vi "WireConnect.vi"(0 "__args":T1) -> (1 "__return":i32, 2 "__errStatus":bool, 3 "__errCode":i32, 4 "__errSource":string)   [LabVIEW 2013]
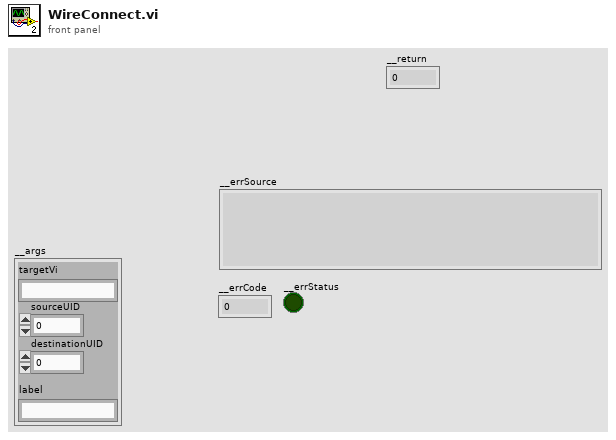
[diagram p1: front panel]
types:
  T1 = cluster{"targetVi":string, "sourceUID":i32, "destinationUID":i32, "label":string}
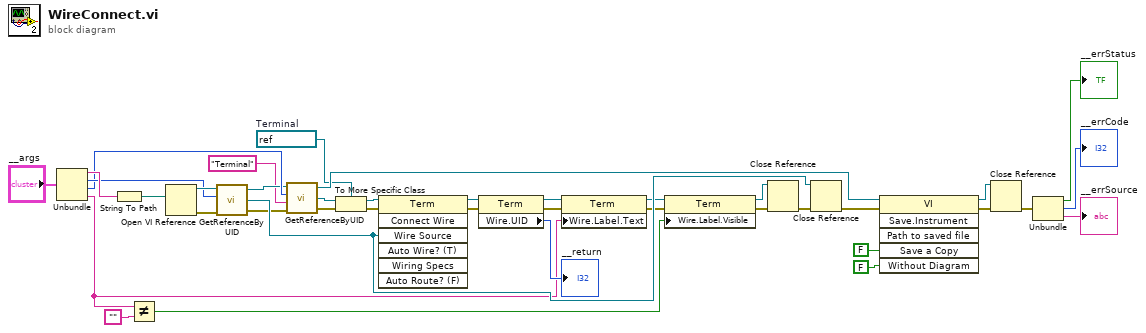
[diagram p0: block diagram]
diagram:
  w11 = refnum<vi> refnum  # Terminal
  n1 = Unbundle("__args") -> ("targetVi"=w28:string, "sourceUID"=w27:i32, "destinationUID"=w26:i32, "label"=w2:string)
  n2 = String To Path(string=w28) -> (path=w35:path)
  n3 = Not Equal?(x=w2, y="") -> (x != y?=w3:bool)
  n4 = Open VI Reference(vi path=w35) -> (vi reference=w34:refnum<vi>, error out=w33:errorcluster)  [unwired: 5 in]
  n5 = call "GetReferenceByUID.vi"("error in (no error)"=w33, "UID"=w27, "targetVI"=w34) -> ("error out"=w13:errorcluster, "refNum"=w14:refnum<vi>, "dup targetVI"=w25:refnum<vi>)  [unwired: 1 in]
  n6 = call "GetReferenceByUID.vi"("error in (no error)"=w13, "objectClass"="Terminal", "UID"=w26, "targetVI"=w25) -> ("error out"=w23:errorcluster, "refNum"=w22:refnum<vi>, "dup targetVI"=w24:refnum<vi>)
  n7 = To More Specific Class(target class=w11, reference=w22, error in=w23) -> (specific class reference=w21:refnum<vi>, error out=w20:errorcluster)
  n8 = invoke class="Term" method="Connect Wire"(reference=w21, error in=w20, "Wire Source"=w14) -> (reference out=w17:refnum<vi>, error out=w15:errorcluster)  [unwired: 4 in, 5 out]
  n9 = property class="Term"(reference=w17, error in=w15) -> (reference out=w9:refnum<vi>, error out=w8:errorcluster, "Wire.UID"=→"__return":i32)
  n10 = property class="Term"(reference=w9, error in=w8, "Wire.Label.Text"=w2) -> (reference out=w4:refnum<vi>, error out=w7:errorcluster)
  n11 = property class="Term"(reference=w4, error in=w7, "Wire.Label.Visible"=w3) -> (reference out=w5:refnum<vi>, error out=w6:errorcluster)
  n12 = Close Reference(reference=w5, error in (no error)=w6) -> (error out=w18:errorcluster)
  n13 = Close Reference(reference=w14, error in (no error)=w18) -> (error out=w19:errorcluster)
  n14 = invoke class="VI" method="Save.Instrument"(reference=w24, error in=w19, "Save a Copy"=FALSE, "Without Diagram"=FALSE) -> (reference out=w32:refnum<vi>, error out=w31:errorcluster)  [unwired: 2 in, 4 out]
  n15 = Close Reference(reference=w32, error in (no error)=w31) -> (error out=w12:errorcluster)
  n16 = Unbundle(w12) -> ("status"=→"__errStatus":bool, "code"=→"__errCode":i32, "source"=→"__errSource":string)
